vi "Connect.vi"(8 "error in (no error)":errorcluster, 11 "Agilent DSO-X 3032A in":refnum<class "Agilent DSO-X 3032A.lvclass">) -> (0 "error out":errorcluster, 3 "Agilent DSO-X 3032A out":refnum<class "Agilent DSO-X 3032A.lvclass">)   [LabVIEW 2014, in "Agilent DSO-X 3032A.lvclass"]
uses:
  Agilent DSO-X 3032A.lvclass
  <vilib>/Utility/error.llb/DialogType.ctl
  Agilent DSO-X 3032A.lvclass/Agilent DSO-X 3032A.ctl
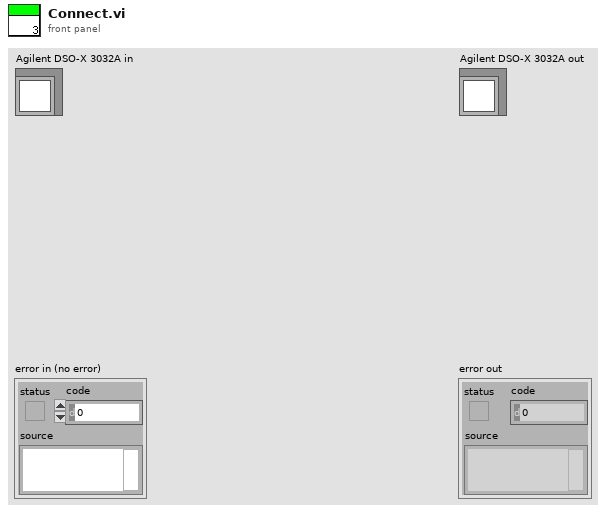
[diagram p1: front panel]
types:
  T1 = typedef "DialogType.ctl" = u16
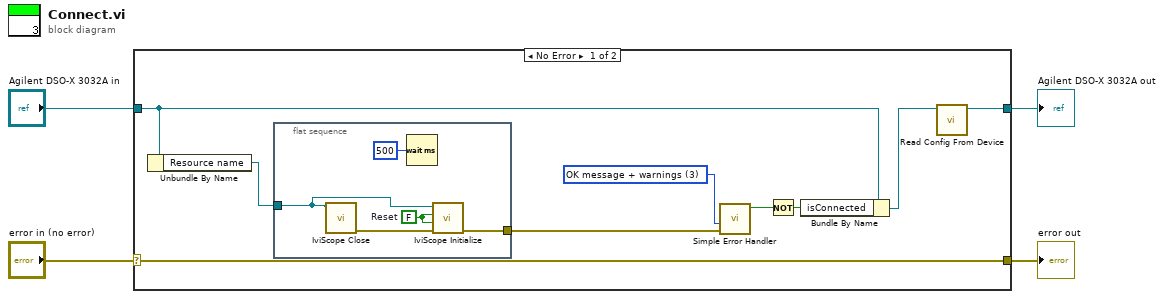
[diagram p0: block diagram]
diagram:
  n1 = case shown="No Error" "error in (no error)" {
    selector: "error in (no error)" -> [w13 w20]
    tunnel: [w13 w20] -> w3
    tunnel: [w7 w19] -> w1
    tunnel: "Agilent DSO-X 3032A in" -> [w9 w19]
    frame No Error {
      w12 = T1 3 items=["no dialog", "OK message", "continue or stop message", "OK message + warnings", "continue/stop + warnings"] ("type of dialog (OK msg:1)")
      n2 = Unbundle By Name(w9) -> ("Resource name"=w5:refnum<k15>)
      n3 = flat-sequence {
        tunnel: [w17] -> w6
        tunnel: w5 -> [w14]
        frame #0 {
          w18 = FALSE  # Reset
          n4 = call <vilib>:"IviScope Close.vi"("instrument handle"=w14) -> ("error out"=w15:errorcluster)  [unwired: 1 in, 9 out]
          n5 = Wait (ms)(milliseconds to wait=u32 500) -> ()  [unwired: 1 out]
          n6 = call <vilib>:"IviScope Initialize.vi"("error in (no error)"=w15, "reset device (True)"=w18, "id query (True)"=w18, "logical name (\"SampleScope\")"=w14) -> ("error out"=w17:errorcluster)  [unwired: 6 in, 1 out]
        }
      }
      n7 = call <vilib>:"Simple Error Handler.vi"("type of dialog (OK msg:1)"=w12, "error in (no error)"=w6) -> ("error?"=w11:bool)  [unwired: 3 in, 4 out]
      n8 = Not(x=w11) -> (.not. x?=w10:bool)
      n9 = Bundle By Name(cluster=w9, "isConnected"=w10) -> (w8:refnum<class "Agilent DSO-X 3032A.lvclass">)
      n10 = call "Read Config From Device.vi"("Agilent DSO-X 3032A in"=w8) -> ("Agilent DSO-X 3032A out"=w7:refnum<class "Agilent DSO-X 3032A.lvclass">)  [unwired: 9 in, 1 out]
    }
    frame Error {
    }
  }
  "error out" <- w3
  "Agilent DSO-X 3032A out" <- w1
